vi "R2_pH Control.vi"(8 "Pump On Time (s)":dbl=7.0, 9 "Reaction Time (s)":dbl=7.0, 10 "pH Set Point":dbl=7.0, 11 "pH Tolerance":dbl=20.0) -> ()   [LabVIEW 2016]
uses:
  R2 Reactor Status v1.ctl
  R2 pH Manual Control.ctl
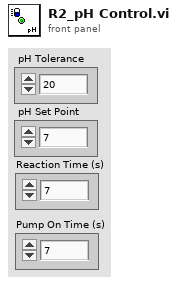
[diagram p1: front panel]
types:
  T1 = typedef "R2Variables.lvlib/R2 Reactor Status v1.ctl" = cluster{"Water Pump":bool, "Media Pump":bool, "Effluent Pump":bool, "Base Pump":bool, "Gas Pump":bool, "Acid Pump":bool, "Air Release Valve":bool, "N2 Valve":bool, "pH":dbl, "DO (mg/L)":dbl, "pH Amp (A)":dbl, "DO Amp (A)":dbl, "Release Flow":dbl, "Compressed Air":dbl, "Reactor Status":sgl, "Air Valve":bool}
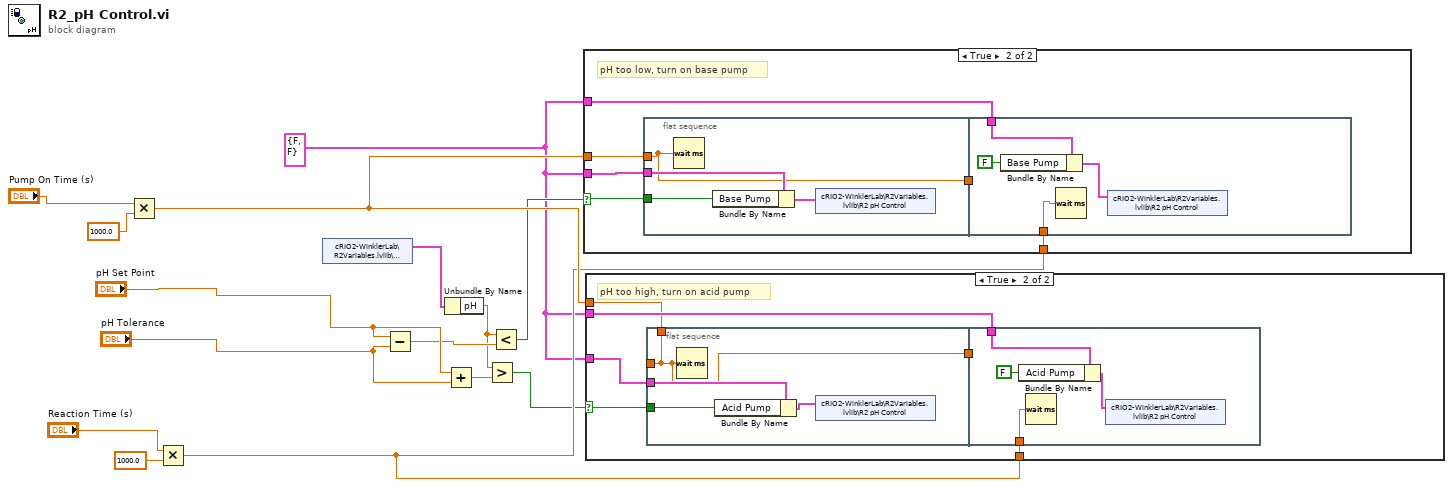
[diagram p0: block diagram]
diagram:
  w1 = cluster{"Acid Pump":bool, "Base Pump":bool} {"Acid Pump"=FALSE, "Base Pump"=FALSE} ("Reactor 2 pH Control")
  n1 = Multiply(x="Pump On Time (s)", y=1000.0) -> (x*y=w9:dbl)
  n2 = Multiply(x="Reaction Time (s)", y=1000.0) -> (x*y=w8:dbl)
  n3 = shared-variable "cRIO2-WinklerLab\\R2Variables.lvlib\\R2Status"() -> (w2:T1)  [unwired: 1 in, 1 out]
  n4 = Subtract(x="pH Set Point", y="pH Tolerance") -> (x-y=w6:dbl)
  n5 = Unbundle By Name(w2) -> ("pH"=w4:dbl)
  n6 = Add(x="pH Set Point", y="pH Tolerance") -> (x+y=w7:dbl)
  n7 = Greater?(x=w4, y=w7) -> (0:w3:bool)
  n8 = Less?(x=w4, y=w6) -> (x < y?=w5:bool)
  n9 = case shown="True" w5 {
    selector: w5 -> [_ w21]
    tunnel: w1 -> [_ w20]
    tunnel: w1 -> [_ w19]
    tunnel: w9 -> [_ w17]
    tunnel: w8 -> [_ w16]
    frame False {
    }
    frame True {
      # "pH too low, turn on base pump"
      n10 = flat-sequence {
        tunnel: w21 -> [w24]
        tunnel: w20 -> [w25]
        tunnel: [w22] -> w18
        tunnel: w17 -> [w22]
        tunnel: w19 -> [w29]
        tunnel: w18 -> [_]
        tunnel: w16 -> [w26]
        frame #0 {
          n11 = Wait (ms)(milliseconds to wait=w22) -> ()  [unwired: 1 out]
          n12 = Bundle By Name(cluster=w25, "Base Pump"=w24) -> (w23:cluster{"Acid Pump":bool, "Base Pump":bool})
          n13 = shared-variable "cRIO2-WinklerLab\\R2Variables.lvlib\\R2 pH Control"(w23) -> ()  [unwired: 1 in, 1 out]
        }
        frame #1 {
          n14 = Bundle By Name(cluster=w29, "Base Pump"=FALSE ("On/Off")) -> (w27:cluster{"Acid Pump":bool, "Base Pump":bool})
          n15 = Wait (ms)(milliseconds to wait=w26) -> ()  [unwired: 1 out]
          n16 = shared-variable "cRIO2-WinklerLab\\R2Variables.lvlib\\R2 pH Control"(w27) -> ()  [unwired: 1 in, 1 out]
        }
      }
    }
  }
  n17 = case shown="True" w3 {
    selector: w3 -> [_ w35]
    tunnel: w1 -> [_ w34]
    tunnel: w1 -> [_ w33]
    tunnel: w9 -> [_ w31]
    tunnel: w8 -> [_ w30]
    frame False {
    }
    frame True {
      # "pH too high, turn on acid pump"
      n18 = flat-sequence {
        tunnel: w35 -> [w39]
        tunnel: [w36] -> _
        tunnel: w34 -> [w38]
        tunnel: [w36] -> w32
        tunnel: w31 -> [w36]
        tunnel: w33 -> [w42]
        tunnel: w32 -> [_]
        tunnel: w30 -> [w40]
        frame #0 {
          n19 = Wait (ms)(milliseconds to wait=w36) -> ()  [unwired: 1 out]
          n20 = Bundle By Name(cluster=w38, "Acid Pump"=w39) -> (w37:cluster{"Acid Pump":bool, "Base Pump":bool})
          n21 = shared-variable "cRIO2-WinklerLab\\R2Variables.lvlib\\R2 pH Control"(w37) -> ()  [unwired: 1 in, 1 out]
        }
        frame #1 {
          n22 = Bundle By Name(cluster=w42, "Acid Pump"=FALSE ("On/Off")) -> (w41:cluster{"Acid Pump":bool, "Base Pump":bool})
          n23 = Wait (ms)(milliseconds to wait=w40) -> ()  [unwired: 1 out]
          n24 = shared-variable "cRIO2-WinklerLab\\R2Variables.lvlib\\R2 pH Control"(w41) -> ()  [unwired: 1 in, 1 out]
        }
      }
    }
  }
